vi "niDTS BT Dut Tx Configure.vi"(0 "Dut Handle in":T2, 5 "niDTS BT DUT Parameters":T1={"Channel"=3, "Pattern"=enum."PN9", "Packet type"=enum."DH1", "Power"=0.0, "Report Period (ms)"=1000.0, "BD Address"=0, "Data Rate"=enum."1", "Number of Packets"=1500, "Packet Length, bytes"=-1} {"BD Address" format="%x"}, 7 "Apply Additional Defaults":bool=TRUE, 11 "error in (no error)":errorcluster) -> (4 "Dut Handle":T2, 15 "error out":errorcluster)   [LabVIEW 2015, in "niDTS BT.lvlib"]
doc: "Set the basic parameters for the WLAN TX Test. \n\nInputs:\n* Apply Additional Defaults. This allows more advanced parameters, which are dependant on the inputs, to have their default values set.\n\nCallbacks:\n* WLAN DUT Additional Defaults\n\nNote: This behavior is expected to be depricated when full parameter sets are passed as inputs and the input dependant defaults are calculated on the top parameter setting level."
uses:
  niDTS BT.lvlib
  Framework/Dut/Includes/niDTS Dut INC Handle.ctl
  Framework/Dut/Objects/BASE_class/niDTS Dut.lvclass
  Includes/niDTS BT DUT INC Parameters.ctl
  Includes/niDTS BT Dut INC Handle.ctl
  Objects/BASE_class/niDTS BT Dut.lvclass
  Framework/Logger/Objects/BASE_class/niDTS Logger.lvclass
  Framework/niDTS Framework.lvlib
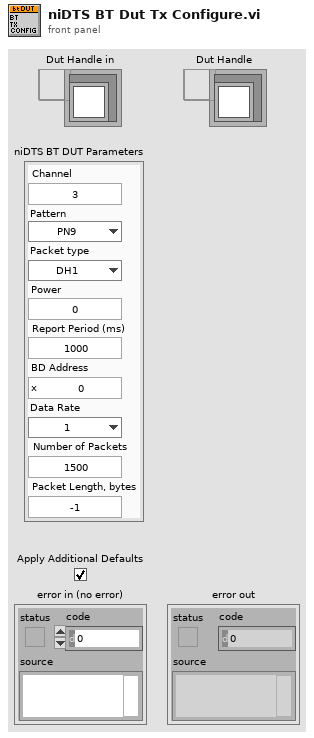
[diagram p1: front panel]
types:
  T1 = typedef "niDTS BT.lvlib/niDTS BT DUT INC Parameters.ctl" = cluster{"Channel":i32, "Pattern":enum16{"0", "1", "01", "00001111", "PN9"}, "Packet type":enum16{"NULL", "POLL", "FHS", "DM1", "DH1", "HV1", "HV2", "HV3", "EV3", "DV", "AUX1", "DM3", "DH3", "EV4", "EV5", "DM5", "DH5", "LE-TP"}, "Power":dbl, "Report Period (ms)":dbl, "BD Address":i64, "Data Rate":enum16{"1", "2", "3"}, "Number of Packets":i32, "Packet Length, bytes":i32}
  T2 = typedef "niDTS Framework.lvlib/niDTS Dut INC Handle.ctl" = refnum<data-value>
  T3 = typedef "niDTS BT.lvlib/niDTS BT Dut INC Handle.ctl" = refnum<data-value>
  T4 = enum16{"NULL", "POLL", "FHS", "DM1", "DH1", "HV1", "HV2", "HV3", "EV3", "DV", "AUX1", "DM3", "DH3", "EV4", "EV5", "DM5", "DH5", "LE-TP"}
  T5 = typedef "niDTS BT.lvlib/niDTS BT INC Standard.ctl" = enum16{"BDR", "EDR", "LE-TP"}
  T6 = typedef "niDTS Framework.lvlib/niDTS Logger INC Handle.ctl" = refnum<data-value>
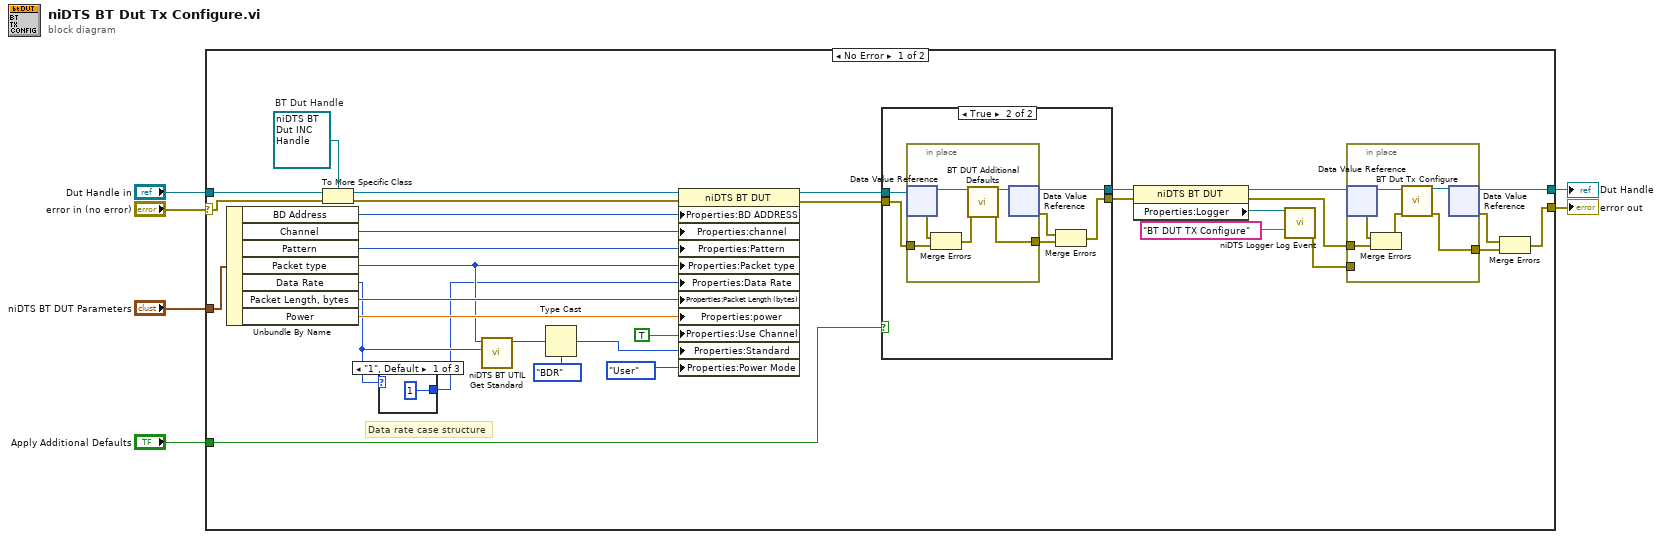
[diagram p0: block diagram]
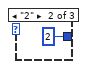
[diagram p2: hidden frame]
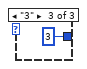
[diagram p3: hidden frame]
diagram:
  n1 = case shown="No Error" "error in (no error)" {
    selector: "error in (no error)" -> [w32 w63]
    tunnel: "Dut Handle in" -> [w39 w64]
    tunnel: "niDTS BT DUT Parameters" -> [w36 _]
    tunnel: "Apply Additional Defaults" -> [w35 _]
    tunnel: [w31 w64] -> w3
    tunnel: [w28 w63] -> w2
    frame No Error {
      w20 = T3 refnum  # BT Dut Handle
      # "Data rate case structure"
      n2 = Unbundle By Name(w36) -> ("BD Address"=w9:i64, "Channel"=w19:i32, "Pattern"=w18:enum16{"0", "1", "01", "00001111", "PN9"}, "Packet type"=w10:T4, "Data Rate"=w8:enum16{"1", "2", "3"}, "Packet Length, bytes"=w17:i32, "Power"=w16:dbl)
      n3 = To More Specific Class(target class=w20, reference=w39, error in=w32) -> (specific class reference=w38:T3, error out=w37:errorcluster)
      n4 = case shown="\"1\", Default" w8 {
        tunnel: [1 2 3] -> w7
        frame "1", Default {
        }
        frame "2" {
        }
        frame "3" {
        }
      }
      n5 = call "niDTS BT UTIL Get Standard.vi"("Data Rate"=w8, "Packet type"=w10) -> ("BT Standard"=w11:T5)  [unwired: 9 in]
      n6 = Type Cast(type=enum16{"BDR", "EDR", "LE"}."BDR" ("Standard"), x=w11) -> (*(type *) &x=w13:enum16{"BDR", "EDR", "LE"})
      n7 = property class="niDTS BT DUT"(reference=w38, error in=w37, "Properties:BD ADDRESS"=w9, "Properties:channel"=w19, "Properties:Pattern"=w18, "Properties:Packet type"=w10, "Properties:Data Rate"=w7, "Properties:Packet Length (bytes)"=w17, "Properties:power"=w16, "Properties:Use Channel"=TRUE ("Use Channel"), "Properties:Standard"=w13, "Properties:Power Mode"=enum16{"Max", "Min", "User"}."User" ("Power Mode")) -> (reference out=w34:T3, error out=w33:errorcluster)
      n8 = case shown="True" w35 {
        tunnel: w34 -> [w50 w56]
        tunnel: w33 -> [w49 w55]
        tunnel: [w50 w52] -> w27
        tunnel: [w49 w51] -> w26
        frame False {
        }
        frame True {
          n9 = in-place {
            in-place-border: [w60] -> w54
            in-place-border: w55 -> [w59]
            n10 = in-place-dvr #1(w56) -> (w62:refnum<class "niDTS BT Dut.lvclass">, w58:errorcluster)
            n11 = Merge Errors(w58, w59) -> (w57:errorcluster)
            n12 = call-dynamic "BT DUT Additional Defaults.vi"("niDTS BT DUT in"=w62, "error in (no error)"=w57) -> ("niDTS BT DUT out"=w61:refnum<class "niDTS BT Dut.lvclass">, "error out"=w60:errorcluster)  [unwired: 12 in]
            n13 = in-place-dvr #1(w61) -> (w52:T3, w53:errorcluster)
          }
          n14 = Merge Errors(w53, w54) -> (w51:errorcluster)
        }
      }
      n15 = property class="niDTS BT DUT"(reference=w27, error in=w26) -> (reference out=w23:T3, error out=w22:errorcluster, "Properties:Logger"=w25:T6)
      n16 = call "niDTS Logger Log Event.vi"("Logger Handle"=w25, "Source/Location"="BT DUT TX Configure") -> ("error out"=w21:errorcluster)  [unwired: 11 in, 2 out]
      n17 = in-place {
        in-place-border: w22 -> [w48]
        in-place-border: [w43] -> w30
        in-place-border: w21 -> [_]
        n18 = in-place-dvr #2(w23) -> (w46:refnum<class "niDTS BT Dut.lvclass">, w47:errorcluster)
        n19 = Merge Errors(w47, w48) -> (w45:errorcluster)
        n20 = call-dynamic "BT Dut Tx Configure.vi"("niDTS BT DUT in"=w46, "error in (no error)"=w45) -> ("niDTS BT DUT out"=w44:refnum<class "niDTS BT Dut.lvclass">, "error out"=w43:errorcluster)  [unwired: 12 in]
        n21 = in-place-dvr #2(w44) -> (w31:T3, w29:errorcluster)
      }
      n22 = Merge Errors(w29, w30) -> (w28:errorcluster)
    }
    frame Error {
    }
  }
  "error out" <- w2
  "Dut Handle" <- w3
